vi "Configure Modulation Waveform Advanced.vi"   [LabVIEW 2012, in "Agilent PSG MXG Series.lvlib"]
doc: "Configures parameters for dual-sine or swept-sine waveform for N5171B, N5172B, N5181B, N5182B."
uses:
  <instrlib>/Agilent PSG MXG Series/Agilent PSG MXG Series.lvlib
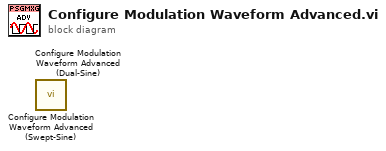
[diagram p0: block diagram]
diagram:
  n1 = call <instrlib>:"Configure Modulation Waveform Advanced (Swept-Sine).vi"() -> ()  [unwired: 14 in, 2 out]
  n2 = call <instrlib>:"Configure Modulation Waveform Advanced (Dual-Sine).vi"() -> ()  [unwired: 14 in, 2 out]
